vi "S4GUI_002.vi"(7 "Tab ObsEng":enum32{"Obs", "CCD modes", "Eng"}(tab)) -> ()   [LabVIEW 2018] (continued)
                    n834 = Not(x=w1534) -> (.not. x?=w1554:bool)
                    n835 = Not(x=w1533) -> (.not. x?=w1553:bool)
                    n836 = Not(x=w1532) -> (.not. x?=w1555:bool)
                    n837 = property on="Image FInal Column 2" class="DigNum (strict)"("Blinking"=w1552) -> ()  [unwired: 2 in, 2 out]
                    n838 = property on="Frame Transfer 2" class="Bool (strict)"("Blinking"=w1550) -> ()  [unwired: 2 in, 2 out]
                    n839 = property on="Vertical Clock Voltage 2" class="Ring (strict)"("Blinking"=w1551) -> ()  [unwired: 2 in, 2 out]
                    n840 = property on="A/D Channel 2" class="DigNum (strict)"("Blinking"=w1549) -> ()  [unwired: 2 in, 2 out]
                    n841 = property on="Image Initial Line 2" class="DigNum (strict)"("Blinking"=w1554) -> ()  [unwired: 2 in, 2 out]
                    n842 = property on="Image Initial Column 2" class="DigNum (strict)"("Blinking"=w1553) -> ()  [unwired: 2 in, 2 out]
                    n843 = property on="Image Final Line 2" class="DigNum (strict)"("Blinking"=w1555) -> ()  [unwired: 2 in, 2 out]
                    n844 = Not(x=w1524) -> (.not. x?=w1545:bool)
                    n845 = Not(x=w1523) -> (.not. x?=w1547:bool)
                    n846 = Not(x=w1522) -> (.not. x?=w1546:bool)
                    n847 = Not(x=w1521) -> (.not. x?=w1548:bool)
                    n848 = Not(x=w1527) -> (.not. x?=w1543:bool)
                    n849 = Not(x=w1526) -> (.not. x?=w1544:bool)
                    n850 = Not(x=w1525) -> (.not. x?=w1542:bool)
                    n851 = property on="Shutter Openning Time 2" class="DigNum (strict)"("Blinking"=w1545) -> ()  [unwired: 2 in, 2 out]
                    n852 = property on="Shutter Closing Time 2" class="DigNum (strict)"("Blinking"=w1547) -> ()  [unwired: 2 in, 2 out]
                    n853 = property on="Vertical Binning 2" class="DigNum (strict)"("Blinking"=w1546) -> ()  [unwired: 2 in, 2 out]
                    n854 = property on="Horizontal Binning 2" class="DigNum (strict)"("Blinking"=w1548) -> ()  [unwired: 2 in, 2 out]
                    n855 = property on="CCD EM Gain 2" class="DigNum (strict)"("Blinking"=w1543) -> ()  [unwired: 2 in, 2 out]
                    n856 = property on="Shutter Mode 2" class="Ring (strict)"("Blinking"=w1544) -> ()  [unwired: 2 in, 2 out]
                    n857 = property on="Shutter TTL 2" class="Ring (strict)"("Blinking"=w1542) -> ()  [unwired: 2 in, 2 out]
                    n858 = Not(x=w1520) -> (.not. x?=w1535:bool)
                    n859 = Not(x=w1516) -> (.not. x?=w1538:bool)
                    n860 = Not(x=w1515) -> (.not. x?=w1536:bool)
                    n861 = Not(x=w1514) -> (.not. x?=w1537:bool)
                    n862 = Not(x=w1519) -> (.not. x?=w1540:bool)
                    n863 = Not(x=w1518) -> (.not. x?=w1539:bool)
                    n864 = Not(x=w1517) -> (.not. x?=w1541:bool)
                    n865 = property on="Acquisition Mode 2" class="Ring (strict)"("Blinking"=w1535) -> ()  [unwired: 2 in, 2 out]
                    n866 = property on="Readout Rate 2" class="Ring (strict)"("Blinking"=w1538) -> ()  [unwired: 2 in, 2 out]
                    n867 = property on="Vertical Shift Speed 2" class="Ring (strict)"("Blinking"=w1536) -> ()  [unwired: 2 in, 2 out]
                    n868 = property on="CCD EM Mode 2" class="Ring (strict)"("Blinking"=w1537) -> ()  [unwired: 2 in, 2 out]
                    n869 = property on="Trigger Mode 2" class="Ring (strict)"("Blinking"=w1540) -> ()  [unwired: 2 in, 2 out]
                    n870 = property on="Read Mode 2" class="Ring (strict)"("Blinking"=w1539) -> ()  [unwired: 2 in, 2 out]
                    n871 = property on="Pre-amplification Gain 2" class="Ring (strict)"("Blinking"=w1541) -> ()  [unwired: 2 in, 2 out]
                  }
                }
                n872 = local read "Cameras Cluster"() -> (w1505:T7)
                n873 = Bundle By Name(cluster=w1505, "Current Configuration.Image Initial Line 2"=w1468, "Current Configuration.Image Initial Column 2"=w1466, "Current Configuration.Image Final Line 2"=w1469, "Current Configuration.Image FInal Column 2"=w1467, "Current Configuration.Vertical Binning 2"=w1472, "Current Configuration.Horizontal Binning 2"=w1503, "Current Configuration.Pre-amplification Gain 2"=w1471, "Current Configuration.CCD EM Gain 2"=w1470, "Current Configuration.Readout Rate 2"=w1465, "Current Configuration.Shutter Openning Time 2"=w1502, "Current Configuration.Shutter Closing Time 2"=w1501, "Current Configuration.Vertical Shift Speed 2"=w1500, "Current Configuration.Read Mode 2"=w1499, "Current Configuration.Vertical Clock Voltage 2"=w1498, "Current Configuration.A/D Channel 2"=w1497, "Current Configuration.Shutter Mode 2"=w1494, "Current Configuration.Shutter TTL 2"=w1495, "Current Configuration.Trigger Mode 2"=w1473, "Current Configuration.Frame Transfer 2"=w1474, "Current Configuration.Acquisition Mode 2"=w1496, "Current Configuration.CCD EM Mode 2"=w1464) -> (w1504:T7)
                n874 = local write "PA2"(w1459) -> ()
                n875 = local write "B2"(w1458) -> ()
                n876 = local write "EA2"(w1460) -> ()
                n877 = local write "SI2"(w1455) -> ()
                n878 = local write "RO2"(w1456) -> ()
                n879 = local write "G2"(w1457) -> ()
                n880 = local write "Cameras Cluster"(w1504) -> ()
                n881 = Compound Arithmetic op=AND(w1479, w1478, w1477, w1476, w1452, w1451, w1475, w1486, w1485, w1484, w1483, w1482, w1481, w1480, w1493, w1492, w1491, w1490, w1489, w1488, w1487) -> (w1450:bool)
                "CCD checked 2" <- w1450
                n882 = disable-structure shown="Disabled" {
                  disable-tunnel: w1450 -> [w1507 _]
                  frame Disabled {
                    n883 = Select(t=u32 1244955, s=w1507, f=u32 16718848) -> (s? t:f=w1510:u32)
                    n884 = property on="CCD checked 2" class="Bool (strict)"("Caption.BG Color"=w1510) -> ()  [unwired: 2 in, 2 out]
                  }
                  frame Enabled {
                  }
                }
                n885 = property on="Acquisition Mode 2" class="Ring (strict)"("DisabledEnum"=w1453) -> ()  [unwired: 2 in, 2 out]
                n886 = property on="Readout Rate 2" class="Ring (strict)"("DisabledEnum"=w1453) -> ()  [unwired: 2 in, 2 out]
                n887 = property on="Vertical Shift Speed 2" class="Ring (strict)"("DisabledEnum"=w1453) -> ()  [unwired: 2 in, 2 out]
                n888 = property on="CCD EM Mode 2" class="Ring (strict)"("DisabledEnum"=w1453) -> ()  [unwired: 2 in, 2 out]
                n889 = property on="Shutter Openning Time 2" class="DigNum (strict)"("DisabledEnum"=w1453) -> ()  [unwired: 2 in, 2 out]
                n890 = property on="Shutter Closing Time 2" class="DigNum (strict)"("DisabledEnum"=w1453) -> ()  [unwired: 2 in, 2 out]
                n891 = property on="Vertical Binning 2" class="DigNum (strict)"("DisabledEnum"=w1453) -> ()  [unwired: 2 in, 2 out]
                n892 = property on="Horizontal Binning 2" class="DigNum (strict)"("DisabledEnum"=w1453) -> ()  [unwired: 2 in, 2 out]
                n893 = property on="Trigger Mode 2" class="Ring (strict)"("DisabledEnum"=w1453) -> ()  [unwired: 2 in, 2 out]
                n894 = property on="Read Mode 2" class="Ring (strict)"("DisabledEnum"=w1453) -> ()  [unwired: 2 in, 2 out]
                n895 = property on="Pre-amplification Gain 2" class="Ring (strict)"("DisabledEnum"=w1453) -> ()  [unwired: 2 in, 2 out]
                n896 = property on="CCD EM Gain 2" class="DigNum (strict)"("DisabledEnum"=w1453) -> ()  [unwired: 2 in, 2 out]
                n897 = property on="Shutter Mode 2" class="Ring (strict)"("DisabledEnum"=w1453) -> ()  [unwired: 2 in, 2 out]
                n898 = property on="Shutter TTL 2" class="Ring (strict)"("DisabledEnum"=w1453) -> ()  [unwired: 2 in, 2 out]
                n899 = property on="Image FInal Column 2" class="DigNum (strict)"("DisabledEnum"=w1453) -> ()  [unwired: 2 in, 2 out]
                n900 = property on="Frame Transfer 2" class="Bool (strict)"("DisabledEnum"=w1453) -> ()  [unwired: 2 in, 2 out]
                n901 = property on="Vertical Clock Voltage 2" class="Ring (strict)"("DisabledEnum"=w1453) -> ()  [unwired: 2 in, 2 out]
                n902 = property on="A/D Channel 2" class="DigNum (strict)"("DisabledEnum"=w1453) -> ()  [unwired: 2 in, 2 out]
                n903 = property on="Image Initial Line 2" class="DigNum (strict)"("DisabledEnum"=w1453) -> ()  [unwired: 2 in, 2 out]
                n904 = property on="Image Initial Column 2" class="DigNum (strict)"("DisabledEnum"=w1453) -> ()  [unwired: 2 in, 2 out]
                n905 = property on="Image Final Line 2" class="DigNum (strict)"("DisabledEnum"=w1453) -> ()  [unwired: 2 in, 2 out]
              }
              frame #17 {
                # "Carrega coluna do Channel 3"
                # "Aba:  Eng->Camera"
                n906 = Unbundle By Name(w1669) -> ("ChannelC_CCD"=w1639:T29, "CHC_Checked Params"=w1654:T14, "ChannelC_Status.connection"=w1632:bool)
                n907 = Unbundle By Name(w1654) -> ("ACQUISITION_MODE"=w1621:bool, "TRIGGER_MODE"=w1620:bool, "READ_MODE"=w1619:bool, "PREAMP"=w1618:bool, "READOUT_RATE"=w1617:bool, "VERTICAL_SHIFT_SPEED"=w1616:bool, "EM_MODE"=w1615:bool, "EM_GAIN"=w1652:bool, "SHUTTER_MODE"=w1651:bool, "SHUTTER_TTL"=w1650:bool, "SHUTTER_OPENING_TIME"=w1649:bool, "SHUTTER_CLOSING_TIME"=w1631:bool, "VBIN"=w1623:bool, "HBIN"=w1622:bool, "INITIAL_LINE"=w1630:bool, "INITIAL_COLUMN"=w1629:bool, "FINAL_LINE"=w1628:bool, "FINAL_COLUMN"=w1627:bool, "FRAME_TRANSFER"=w1626:bool, "VERTICAL_CLOCK_VOLTAGE"=w1625:bool, "AD_CHANNEL"=w1624:bool)
                n908 = case shown="True" w1632 {
                  tunnel: w1639 -> [_ w1722]
                  tunnel: [w1715 w1721] -> w1638
                  tunnel: [w1715 w1720] -> w1637
                  tunnel: [w1715 w1719] -> w1636
                  tunnel: [w1715 w1718] -> w1635
                  tunnel: [w1715 w1717] -> w1634
                  tunnel: [w1715 w1716] -> w1633
                  frame False {
                    w1715 = ""
                  }
                  frame True {
                    n909 = stacked-sequence "Atualizacao dos indicadores inferiores do CANAL C da tela principal" {
                      tunnel: w1722 -> [w1737 w1740 w1745 w1754 w1757 w1761]
                      tunnel: [w1723 _ _ _ _ _] -> w1721
                      tunnel: [_ w1738 _ _ _ _] -> w1720
                      tunnel: [_ _ w1743 _ _ _] -> w1719
                      tunnel: [_ _ _ w1748 _ _] -> w1718
                      tunnel: [_ _ _ _ w1755 _] -> w1717
                      tunnel: [_ _ _ _ _ w1758] -> w1716
                      frame #0 {
                        # "SubImage"
                        n910 = Unbundle By Name(w1737) -> ("INITIAL_LINE"=w1735:u16, "FINAL_LINE"=w1734:u16, "INITIAL_COLUMN"=w1733:u16, "FINAL_COLUMN"=w1732:u16)
                        n911 = Number To Decimal String(number=w1735) -> (decimal integer string=w1731:string)  [unwired: 1 in]
                        n912 = Number To Decimal String(number=w1734) -> (decimal integer string=w1729:string)  [unwired: 1 in]
                        n913 = Number To Decimal String(number=w1733) -> (decimal integer string=w1727:string)  [unwired: 1 in]
                        n914 = Number To Decimal String(number=w1732) -> (decimal integer string=w1725:string)  [unwired: 1 in]
                        n915 = Concatenate Strings("[", w1731, ":", w1729, ",", w1727, ":", w1725, "]") -> (w1723:string)
                      }
                      frame #1 {
                        # "Em Active"
                        n916 = Unbundle By Name(w1740) -> ("EM_MODE"=w1739:u8)
                        n917 = case shown="0, Default" w1739 {
                          tunnel: ["Electron M." ("EmActive1") "Convent." ("EmActive1")] -> w1738
                          frame 0, Default {
                          }
                          frame 1 {
                          }
                        }
                      }
                      frame #2 {
                        # "Pre Amp"
                        n918 = Unbundle By Name(w1745) -> ("PREAMP"=w1744:u8)
                        n919 = case shown="1" w1744 {
                          tunnel: ["Gain 1" ("EmActive1") "Gain 2" ("EmActive1")] -> w1743
                          frame 0, Default {
                          }
                          frame 1 {
                          }
                        }
                      }
                      frame #3 {
                        # "Binning"
                        n920 = Unbundle By Name(w1754) -> ("VBIN"=w1753:u16, "HBIN"=w1752:u16)
                        n921 = Number To Decimal String(number=w1752) -> (decimal integer string=w1749:string)  [unwired: 1 in]
                        n922 = Number To Decimal String(number=w1753) -> (decimal integer string=w1751:string)  [unwired: 1 in]
                        n923 = Concatenate Strings(w1751, "x", w1749) -> (w1748:string)
                      }
                      frame #4 {
                        # "Gain"
                        n924 = Unbundle By Name(w1757) -> ("EM_GAIN"=w1756:u16)
                        n925 = Number To Decimal String(number=w1756) -> (decimal integer string=w1755:string)  [unwired: 1 in]
                      }
                      frame #5 {
                        # "Readout"
                        n926 = Unbundle By Name(w1761) -> ("EM_MODE"=w1760:u8, "READOUT_RATE"=w1759:u8)
                        n927 = case shown="0, Default" w1760 {
                          tunnel: w1759 -> [w1763 w1769]
                          tunnel: [w1762 w1768] -> w1758
                          frame 0, Default {
                            n928 = case shown="3" w1763 {
                              tunnel: ["30 MHz" ("EmActive1") "20 MHz" ("EmActive1") "10 MHz" ("EmActive1") "1 MHz" ("EmActive1")] -> w1762
                              frame 0, Default {
                              }
                              frame 1 {
                              }
                              frame 2 {
                              }
                              frame 3 {
                              }
                            }
                          }
                          frame 1 {
                            n929 = case shown="1" w1769 {
                              tunnel: ["1 MHz" ("EmActive1") "0.1 MHz" ("EmActive1")] -> w1768
                              frame 0, Default {
                              }
                              frame 1 {
                              }
                            }
                          }
                        }
                      }
                    }
                  }
                }
                n930 = Unbundle By Name(w1639) -> ("INITIAL_LINE"=w1644:u16, "INITIAL_COLUMN"=w1642:u16, "FINAL_LINE"=w1645:u16, "FINAL_COLUMN"=w1643:u16, "VBIN"=w1648:u16, "HBIN"=w1666:u16, "PREAMP"=w1647:u8, "EM_GAIN"=w1646:u16, "READOUT_RATE"=w1641:u8, "SHUTTER_OPENNING_TIME"=w1665:u16, "SHUTTER_CLOSING_TIME"=w1664:u16, "VERTICAL_SHIFT_SPEED"=w1663:u8, "READ_MODE"=w1662:u8, "VERTICAL_CLOCK_VOLTAGE"=w1661:u8, "AD_CHANNEL"=w1660:u32, "SHUTTER_MODE"=w1655:u8, "SHUTTER_TTL"=w1656:u8, "TRIGGER_MODE"=w1657:u8, "FRAME_TRANSFER"=w1658:bool, "ACQUISITION_MODE"=w1659:u8, "EM_MODE"=w1640:u8)
                n931 = local read "CH3 on"() -> (w1614:bool)
                n932 = case shown="True" w1614 {
                  tunnel: w1652 -> [_ w1695]
                  tunnel: w1651 -> [_ w1694]
                  tunnel: w1650 -> [_ w1692]
                  tunnel: w1649 -> [_ w1691]
                  tunnel: w1631 -> [_ w1690]
                  tunnel: w1630 -> [_ w1689]
                  tunnel: w1629 -> [_ w1688]
                  tunnel: w1628 -> [_ w1687]
                  tunnel: w1627 -> [_ w1686]
                  tunnel: w1626 -> [_ w1685]
                  tunnel: w1625 -> [_ w1684]
                  tunnel: w1624 -> [_ w1683]
                  tunnel: w1623 -> [_ w1682]
                  tunnel: w1622 -> [_ w1681]
                  tunnel: w1621 -> [_ w1680]
                  tunnel: w1620 -> [_ w1679]
                  tunnel: w1619 -> [_ w1678]
                  tunnel: w1618 -> [_ w1677]
                  tunnel: w1617 -> [_ w1676]
                  tunnel: w1616 -> [_ w1675]
                  tunnel: w1615 -> [_ w1674]
                  tunnel: [T12."Disabled and Grayed Out" ("Disabled") T12."Enabled" ("Disabled")] -> w1613
                  frame False {
                    w1670 = FALSE
                    n933 = property on="Image Initial Line 3" class="DigNum (strict)"("Blinking"=w1670) -> ()  [unwired: 2 in, 2 out]
                    n934 = property on="Image Initial Column 3" class="DigNum (strict)"("Blinking"=w1670) -> ()  [unwired: 2 in, 2 out]
                    n935 = property on="Image Final Line 3" class="DigNum (strict)"("Blinking"=w1670) -> ()  [unwired: 2 in, 2 out]
                    n936 = property on="Image FInal Column 3" class="DigNum (strict)"("Blinking"=w1670) -> ()  [unwired: 2 in, 2 out]
                    n937 = property on="Frame Transfer 3" class="Bool (strict)"("Blinking"=w1670) -> ()  [unwired: 2 in, 2 out]
                    n938 = property on="Vertical Clock Voltage 3" class="Ring (strict)"("Blinking"=w1670) -> ()  [unwired: 2 in, 2 out]
                    n939 = property on="A/D Channel 3" class="DigNum (strict)"("Blinking"=w1670) -> ()  [unwired: 2 in, 2 out]
                    n940 = property on="CCD EM Gain 3" class="DigNum (strict)"("Blinking"=w1670) -> ()  [unwired: 2 in, 2 out]
                    n941 = property on="Shutter Mode 3" class="Ring (strict)"("Blinking"=w1670) -> ()  [unwired: 2 in, 2 out]
                    n942 = property on="Shutter TTL 3" class="Ring (strict)"("Blinking"=w1670) -> ()  [unwired: 2 in, 2 out]
                    n943 = property on="Shutter Openning Time 3" class="DigNum (strict)"("Blinking"=w1670) -> ()  [unwired: 2 in, 2 out]
                    n944 = property on="Shutter Closing Time 3" class="DigNum (strict)"("Blinking"=w1670) -> ()  [unwired: 2 in, 2 out]
                    n945 = property on="Vertical Binning 3" class="DigNum (strict)"("Blinking"=w1670) -> ()  [unwired: 2 in, 2 out]
                    n946 = property on="Horizontal Binning 3" class="DigNum (strict)"("Blinking"=w1670) -> ()  [unwired: 2 in, 2 out]
                    n947 = property on="Acquisition Mode 3" class="Ring (strict)"("Blinking"=w1670) -> ()  [unwired: 2 in, 2 out]
                    n948 = property on="Vertical Shift Speed 3" class="Ring (strict)"("Blinking"=w1670) -> ()  [unwired: 2 in, 2 out]
                    n949 = property on="Trigger Mode 3" class="Ring (strict)"("Blinking"=w1670) -> ()  [unwired: 2 in, 2 out]
                    n950 = property on="Read Mode 3" class="Ring (strict)"("Blinking"=w1670) -> ()  [unwired: 2 in, 2 out]
                    n951 = property on="Readout Rate 3" class="Ring (strict)"("Blinking"=w1670) -> ()  [unwired: 2 in, 2 out]
                    n952 = property on="CCD EM Mode 3" class="Ring (strict)"("Blinking"=w1670) -> ()  [unwired: 2 in, 2 out]
                    n953 = property on="Pre-amplification Gain 3" class="Ring (strict)"("Blinking"=w1670) -> ()  [unwired: 2 in, 2 out]
                  }
                  frame True {
                    n954 = Not(x=w1689) -> (.not. x?=w1672:bool)
                    n955 = Not(x=w1688) -> (.not. x?=w1713:bool)
                    n956 = Not(x=w1687) -> (.not. x?=w1714:bool)
                    n957 = Not(x=w1686) -> (.not. x?=w1712:bool)
                    n958 = Not(x=w1685) -> (.not. x?=w1710:bool)
                    n959 = Not(x=w1684) -> (.not. x?=w1711:bool)
                    n960 = Not(x=w1683) -> (.not. x?=w1709:bool)
                    n961 = property on="Image FInal Column 3" class="DigNum (strict)"("Blinking"=w1712) -> ()  [unwired: 2 in, 2 out]
                    n962 = property on="Frame Transfer 3" class="Bool (strict)"("Blinking"=w1710) -> ()  [unwired: 2 in, 2 out]
                    n963 = property on="Vertical Clock Voltage 3" class="Ring (strict)"("Blinking"=w1711) -> ()  [unwired: 2 in, 2 out]
                    n964 = property on="Image Initial Line 3" class="DigNum (strict)"("Blinking"=w1672) -> ()  [unwired: 2 in, 2 out]
                    n965 = property on="Image Initial Column 3" class="DigNum (strict)"("Blinking"=w1713) -> ()  [unwired: 2 in, 2 out]
                    n966 = property on="Image Final Line 3" class="DigNum (strict)"("Blinking"=w1714) -> ()  [unwired: 2 in, 2 out]
                    n967 = property on="A/D Channel 3" class="DigNum (strict)"("Blinking"=w1709) -> ()  [unwired: 2 in, 2 out]
                    n968 = Not(x=w1691) -> (.not. x?=w1705:bool)
                    n969 = Not(x=w1690) -> (.not. x?=w1707:bool)
                    n970 = Not(x=w1682) -> (.not. x?=w1706:bool)
                    n971 = Not(x=w1681) -> (.not. x?=w1708:bool)
                    n972 = Not(x=w1695) -> (.not. x?=w1704:bool)
                    n973 = Not(x=w1694) -> (.not. x?=w1693:bool)
                    n974 = Not(x=w1692) -> (.not. x?=w1703:bool)
                    n975 = property on="Shutter Openning Time 3" class="DigNum (strict)"("Blinking"=w1705) -> ()  [unwired: 2 in, 2 out]
                    n976 = property on="Shutter Closing Time 3" class="DigNum (strict)"("Blinking"=w1707) -> ()  [unwired: 2 in, 2 out]
                    n977 = property on="Vertical Binning 3" class="DigNum (strict)"("Blinking"=w1706) -> ()  [unwired: 2 in, 2 out]
                    n978 = property on="Horizontal Binning 3" class="DigNum (strict)"("Blinking"=w1708) -> ()  [unwired: 2 in, 2 out]
                    n979 = property on="CCD EM Gain 3" class="DigNum (strict)"("Blinking"=w1704) -> ()  [unwired: 2 in, 2 out]
                    n980 = property on="Shutter Mode 3" class="Ring (strict)"("Blinking"=w1693) -> ()  [unwired: 2 in, 2 out]
                    n981 = property on="Shutter TTL 3" class="Ring (strict)"("Blinking"=w1703) -> ()  [unwired: 2 in, 2 out]
                    n982 = Not(x=w1680) -> (.not. x?=w1696:bool)
                    n983 = Not(x=w1676) -> (.not. x?=w1699:bool)
                    n984 = Not(x=w1675) -> (.not. x?=w1697:bool)
                    n985 = Not(x=w1674) -> (.not. x?=w1698:bool)
                    n986 = Not(x=w1679) -> (.not. x?=w1701:bool)
                    n987 = Not(x=w1678) -> (.not. x?=w1700:bool)
                    n988 = Not(x=w1677) -> (.not. x?=w1702:bool)
                    n989 = property on="Acquisition Mode 3" class="Ring (strict)"("Blinking"=w1696) -> ()  [unwired: 2 in, 2 out]
                    n990 = property on="Readout Rate 3" class="Ring (strict)"("Blinking"=w1699) -> ()  [unwired: 2 in, 2 out]
                    n991 = property on="Vertical Shift Speed 3" class="Ring (strict)"("Blinking"=w1697) -> ()  [unwired: 2 in, 2 out]
                    n992 = property on="CCD EM Mode 3" class="Ring (strict)"("Blinking"=w1698) -> ()  [unwired: 2 in, 2 out]
                    n993 = property on="Trigger Mode 3" class="Ring (strict)"("Blinking"=w1701) -> ()  [unwired: 2 in, 2 out]
                    n994 = property on="Read Mode 3" class="Ring (strict)"("Blinking"=w1700) -> ()  [unwired: 2 in, 2 out]
                    n995 = property on="Pre-amplification Gain 3" class="Ring (strict)"("Blinking"=w1702) -> ()  [unwired: 2 in, 2 out]
                  }
                }
                n996 = local write "RO3"(w1633) -> ()
                n997 = local write "B3"(w1635) -> ()
                n998 = local write "PA3"(w1636) -> ()
                n999 = local write "EA3"(w1637) -> ()
                n1000 = local write "G3"(w1634) -> ()
                n1001 = local write "SI3"(w1638) -> ()
                n1002 = local read "Cameras Cluster"() -> (w1668:T7)
                n1003 = Bundle By Name(cluster=w1668, "Current Configuration.Image Initial Line 3"=w1644, "Current Configuration.Image Initial Column 3"=w1642, "Current Configuration.Image Final Line 3"=w1645, "Current Configuration.Image FInal Column 3"=w1643, "Current Configuration.Vertical Binning 3"=w1648, "Current Configuration.Horizontal Binning 3"=w1666, "Current Configuration.Pre-amplification Gain 3"=w1647, "Current Configuration.CCD EM Gain 3"=w1646, "Current Configuration.Readout Rate 3"=w1641, "Current Configuration.Shutter Openning Time 3"=w1665, "Current Configuration.Shutter Closing Time 3"=w1664, "Current Configuration.Vertical Shift Speed 3"=w1663, "Current Configuration.Read Mode 3"=w1662, "Current Configuration.Vertical Clock Voltage 3"=w1661, "Current Configuration.A/D Channel 3"=w1660, "Current Configuration.Shutter Mode 3"=w1655, "Current Configuration.Shutter TTL 3"=w1656, "Current Configuration.Trigger Mode 3"=w1657, "Current Configuration.Frame Transfer 3"=w1658, "Current Configuration.Acquisition Mode 3"=w1659, "Current Configuration.CCD EM Mode 3"=w1640) -> (w1667:T7)
                n1004 = local write "Cameras Cluster"(w1667) -> ()
                n1005 = Compound Arithmetic op=AND(w1621, w1620, w1619, w1618, w1617, w1616, w1615, w1652, w1651, w1650, w1649, w1631, w1623, w1622, w1630, w1629, w1628, w1627, w1626, w1625, w1624) -> (→"CCD checked 3":bool)
                n1006 = property on="Image Initial Line 3" class="DigNum (strict)"("DisabledEnum"=w1613) -> ()  [unwired: 2 in, 2 out]
                n1007 = property on="Image Initial Column 3" class="DigNum (strict)"("DisabledEnum"=w1613) -> ()  [unwired: 2 in, 2 out]
                n1008 = property on="Image Final Line 3" class="DigNum (strict)"("DisabledEnum"=w1613) -> ()  [unwired: 2 in, 2 out]
                n1009 = property on="Image FInal Column 3" class="DigNum (strict)"("DisabledEnum"=w1613) -> ()  [unwired: 2 in, 2 out]
                n1010 = property on="Frame Transfer 3" class="Bool (strict)"("DisabledEnum"=w1613) -> ()  [unwired: 2 in, 2 out]
                n1011 = property on="Horizontal Binning 3" class="DigNum (strict)"("DisabledEnum"=w1613) -> ()  [unwired: 2 in, 2 out]
                n1012 = property on="Vertical Clock Voltage 3" class="Ring (strict)"("DisabledEnum"=w1613) -> ()  [unwired: 2 in, 2 out]
                n1013 = property on="CCD EM Gain 3" class="DigNum (strict)"("DisabledEnum"=w1613) -> ()  [unwired: 2 in, 2 out]
                n1014 = property on="Shutter Mode 3" class="Ring (strict)"("DisabledEnum"=w1613) -> ()  [unwired: 2 in, 2 out]
                n1015 = property on="Shutter Openning Time 3" class="DigNum (strict)"("DisabledEnum"=w1613) -> ()  [unwired: 2 in, 2 out]
                n1016 = property on="Shutter Closing Time 3" class="DigNum (strict)"("DisabledEnum"=w1613) -> ()  [unwired: 2 in, 2 out]
                n1017 = property on="Vertical Binning 3" class="DigNum (strict)"("DisabledEnum"=w1613) -> ()  [unwired: 2 in, 2 out]
                n1018 = property on="Shutter TTL 3" class="Ring (strict)"("DisabledEnum"=w1613) -> ()  [unwired: 2 in, 2 out]
                n1019 = property on="Pre-amplification Gain 3" class="Ring (strict)"("DisabledEnum"=w1613) -> ()  [unwired: 2 in, 2 out]
                n1020 = property on="Acquisition Mode 3" class="Ring (strict)"("DisabledEnum"=w1613) -> ()  [unwired: 2 in, 2 out]
                n1021 = property on="Trigger Mode 3" class="Ring (strict)"("DisabledEnum"=w1613) -> ()  [unwired: 2 in, 2 out]
                n1022 = property on="Read Mode 3" class="Ring (strict)"("DisabledEnum"=w1613) -> ()  [unwired: 2 in, 2 out]
                n1023 = property on="Readout Rate 3" class="Ring (strict)"("DisabledEnum"=w1613) -> ()  [unwired: 2 in, 2 out]
                n1024 = property on="A/D Channel 3" class="DigNum (strict)"("DisabledEnum"=w1613) -> ()  [unwired: 2 in, 2 out]
                n1025 = property on="Vertical Shift Speed 3" class="Ring (strict)"("DisabledEnum"=w1613) -> ()  [unwired: 2 in, 2 out]
                n1026 = property on="CCD EM Mode 3" class="Ring (strict)"("DisabledEnum"=w1613) -> ()  [unwired: 2 in, 2 out]
              }
              frame #18 {
                # "Carrega coluna do Channel 4"
                # "Aba:  Eng->Camera"
                n1027 = Unbundle By Name(w1828) -> ("ChannelD_CCD"=w1781:T29, "CHD_Checked Params"=w1813:T14, "ChannelD_Status.connection"=w1780:bool)
                n1028 = Unbundle By Name(w1813) -> ("ACQUISITION_MODE"=w1797:bool, "TRIGGER_MODE"=w1796:bool, "READ_MODE"=w1795:bool, "PREAMP"=w1794:bool, "READOUT_RATE"=w1793:bool, "VERTICAL_SHIFT_SPEED"=w1792:bool, "EM_MODE"=w1791:bool, "EM_GAIN"=w1804:bool, "SHUTTER_MODE"=w1803:bool, "SHUTTER_TTL"=w1802:bool, "SHUTTER_OPENING_TIME"=w1801:bool, "SHUTTER_CLOSING_TIME"=w1800:bool, "VBIN"=w1799:bool, "HBIN"=w1798:bool, "INITIAL_LINE"=w1811:bool, "INITIAL_COLUMN"=w1810:bool, "FINAL_LINE"=w1809:bool, "FINAL_COLUMN"=w1808:bool, "FRAME_TRANSFER"=w1807:bool, "VERTICAL_CLOCK_VOLTAGE"=w1806:bool, "AD_CHANNEL"=w1805:bool)
                n1029 = case shown="True" w1780 {
                  tunnel: w1781 -> [_ w1881]
                  tunnel: [w1874 w1880] -> w1779
                  tunnel: [w1874 w1879] -> w1778
                  tunnel: [w1874 w1878] -> w1777
                  tunnel: [w1874 w1877] -> w1776
                  tunnel: [w1874 w1876] -> w1775
                  tunnel: [w1874 w1875] -> w1774
                  frame False {
                    w1874 = ""
                  }
                  frame True {
                    n1030 = stacked-sequence "Atualizacao dos indicadores inferiores do CANAL D da tela principal" {
                      tunnel: w1881 -> [w1896 w1899 w1904 w1913 w1916 w1920]
                      tunnel: [w1882 _ _ _ _ _] -> w1880
                      tunnel: [_ w1897 _ _ _ _] -> w1879
                      tunnel: [_ _ w1902 _ _ _] -> w1878
                      tunnel: [_ _ _ w1907 _ _] -> w1877
                      tunnel: [_ _ _ _ w1914 _] -> w1876
                      tunnel: [_ _ _ _ _ w1917] -> w1875
                      frame #0 {
                        # "SubImage"
                        n1031 = Unbundle By Name(w1896) -> ("INITIAL_LINE"=w1894:u16, "FINAL_LINE"=w1893:u16, "INITIAL_COLUMN"=w1892:u16, "FINAL_COLUMN"=w1891:u16)
                        n1032 = Number To Decimal String(number=w1894) -> (decimal integer string=w1890:string)  [unwired: 1 in]
                        n1033 = Number To Decimal String(number=w1893) -> (decimal integer string=w1888:string)  [unwired: 1 in]
                        n1034 = Number To Decimal String(number=w1892) -> (decimal integer string=w1886:string)  [unwired: 1 in]
                        n1035 = Number To Decimal String(number=w1891) -> (decimal integer string=w1884:string)  [unwired: 1 in]
                        n1036 = Concatenate Strings("[", w1890, ":", w1888, ",", w1886, ":", w1884, "]") -> (w1882:string)
                      }
                      frame #1 {
                        # "Em Active"
                        n1037 = Unbundle By Name(w1899) -> ("EM_MODE"=w1898:u8)
                        n1038 = case shown="0, Default" w1898 {
                          tunnel: ["Electron M." ("EmActive1") "Convent." ("EmActive1")] -> w1897
                          frame 0, Default {
                          }
                          frame 1 {
                          }
                        }
                      }
                      frame #2 {
                        # "Pre Amp"
                        n1039 = Unbundle By Name(w1904) -> ("PREAMP"=w1903:u8)
                        n1040 = case shown="1" w1903 {
                          tunnel: ["Gain 1" ("EmActive1") "Gain 2" ("EmActive1")] -> w1902
                          frame 0, Default {
                          }
                          frame 1 {
                          }
                        }
                      }
                      frame #3 {
                        # "Binning"
                        n1041 = Unbundle By Name(w1913) -> ("VBIN"=w1912:u16, "HBIN"=w1911:u16)
                        n1042 = Number To Decimal String(number=w1911) -> (decimal integer string=w1908:string)  [unwired: 1 in]
                        n1043 = Number To Decimal String(number=w1912) -> (decimal integer string=w1910:string)  [unwired: 1 in]
                        n1044 = Concatenate Strings(w1910, "x", w1908) -> (w1907:string)
                      }
                      frame #4 {
                        # "Gain"
                        n1045 = Unbundle By Name(w1916) -> ("EM_GAIN"=w1915:u16)
                        n1046 = Number To Decimal String(number=w1915) -> (decimal integer string=w1914:string)  [unwired: 1 in]
                      }
                      frame #5 {
                        # "Readout"
                        n1047 = Unbundle By Name(w1920) -> ("EM_MODE"=w1919:u8, "READOUT_RATE"=w1918:u8)
                        n1048 = case shown="0, Default" w1919 {
                          tunnel: w1918 -> [w1922 w1928]
                          tunnel: [w1921 w1927] -> w1917
                          frame 0, Default {
                            n1049 = case shown="3" w1922 {
                              tunnel: ["30 MHz" ("EmActive1") "20 MHz" ("EmActive1") "10 MHz" ("EmActive1") "1 MHz" ("EmActive1")] -> w1921
                              frame 0, Default {
                              }
                              frame 1 {
                              }
                              frame 2 {
                              }
                              frame 3 {
                              }
                            }
                          }
                          frame 1 {
                            n1050 = case shown="0, Default" w1928 {
                              tunnel: ["1 MHz" ("EmActive1") "0.1 MHz" ("EmActive1")] -> w1927
                              frame 0, Default {
                              }
                              frame 1 {
                              }
                            }
                          }
                        }
                      }
                    }
                  }
                }
                n1051 = Unbundle By Name(w1781) -> ("INITIAL_LINE"=w1786:u16, "INITIAL_COLUMN"=w1784:u16, "FINAL_LINE"=w1787:u16, "FINAL_COLUMN"=w1785:u16, "VBIN"=w1790:u16, "HBIN"=w1825:u16, "PREAMP"=w1789:u8, "EM_GAIN"=w1788:u16, "READOUT_RATE"=w1783:u8, "SHUTTER_OPENNING_TIME"=w1824:u16, "SHUTTER_CLOSING_TIME"=w1823:u16, "VERTICAL_SHIFT_SPEED"=w1822:u8, "READ_MODE"=w1821:u8, "VERTICAL_CLOCK_VOLTAGE"=w1820:u8, "AD_CHANNEL"=w1819:u32, "SHUTTER_MODE"=w1814:u8, "SHUTTER_TTL"=w1815:u8, "TRIGGER_MODE"=w1816:u8, "FRAME_TRANSFER"=w1817:bool, "ACQUISITION_MODE"=w1818:u8, "EM_MODE"=w1782:u8)
                n1052 = local read "CH4 on"() -> (w1773:bool)
                n1053 = case shown="False" w1773 {
                  tunnel: w1811 -> [_ w1853]
                  tunnel: w1810 -> [_ w1852]
                  tunnel: w1809 -> [_ w1851]
                  tunnel: w1808 -> [_ w1850]
                  tunnel: w1807 -> [_ w1849]
                  tunnel: w1806 -> [_ w1848]
                  tunnel: w1805 -> [_ w1847]
                  tunnel: w1804 -> [_ w1846]
                  tunnel: w1803 -> [_ w1845]
                  tunnel: w1802 -> [_ w1844]
                  tunnel: w1801 -> [_ w1843]
                  tunnel: w1800 -> [_ w1842]
                  tunnel: w1799 -> [_ w1841]
                  tunnel: w1798 -> [_ w1840]
                  tunnel: w1797 -> [_ w1839]
                  tunnel: w1796 -> [_ w1838]
                  tunnel: w1795 -> [_ w1837]
                  tunnel: w1794 -> [_ w1835]
                  tunnel: w1793 -> [_ w1834]
                  tunnel: w1792 -> [_ w1833]
                  tunnel: w1791 -> [_ w1832]
                  tunnel: [T12."Disabled and Grayed Out" ("Disabled") T12."Enabled" ("Disabled")] -> w1772
                  frame False {
                    w1830 = FALSE ("Blinking")
                    n1054 = property on="Image FInal Column 4" class="DigNum (strict)"("Blinking"=w1830) -> ()  [unwired: 2 in, 2 out]
                    n1055 = property on="Frame Transfer 4" class="Bool (strict)"("Blinking"=w1830) -> ()  [unwired: 2 in, 2 out]
                    n1056 = property on="Vertical Clock Voltage 4" class="Ring (strict)"("Blinking"=w1830) -> ()  [unwired: 2 in, 2 out]
                    n1057 = property on="A/D Channel 4" class="DigNum (strict)"("Blinking"=w1830) -> ()  [unwired: 2 in, 2 out]
                    n1058 = property on="Image Initial Line 4" class="DigNum (strict)"("Blinking"=w1830) -> ()  [unwired: 2 in, 2 out]
                    n1059 = property on="Image Initial Column 4" class="DigNum (strict)"("Blinking"=w1830) -> ()  [unwired: 2 in, 2 out]
                    n1060 = property on="Image Final Line 4" class="DigNum (strict)"("Blinking"=w1830) -> ()  [unwired: 2 in, 2 out]
                    n1061 = property on="Shutter Openning Time 4" class="DigNum (strict)"("Blinking"=w1830) -> ()  [unwired: 2 in, 2 out]
                    n1062 = property on="Shutter Closing Time 4" class="DigNum (strict)"("Blinking"=w1830) -> ()  [unwired: 2 in, 2 out]
                    n1063 = property on="Vertical Binning 4" class="DigNum (strict)"("Blinking"=w1830) -> ()  [unwired: 2 in, 2 out]
                    n1064 = property on="Horizontal Binning 4" class="DigNum (strict)"("Blinking"=w1830) -> ()  [unwired: 2 in, 2 out]
                    n1065 = property on="CCD EM Gain 4" class="DigNum (strict)"("Blinking"=w1830) -> ()  [unwired: 2 in, 2 out]
                    n1066 = property on="Shutter Mode 4" class="Ring (strict)"("Blinking"=w1830) -> ()  [unwired: 2 in, 2 out]
                    n1067 = property on="Shutter TTL 4" class="Ring (strict)"("Blinking"=w1830) -> ()  [unwired: 2 in, 2 out]
                    n1068 = property on="Acquisition Mode 4" class="Ring (strict)"("Blinking"=w1830) -> ()  [unwired: 2 in, 2 out]
                    n1069 = property on="Readout Rate 4" class="Ring (strict)"("Blinking"=w1830) -> ()  [unwired: 2 in, 2 out]
                    n1070 = property on="Vertical Shift Speed 4" class="Ring (strict)"("Blinking"=w1830) -> ()  [unwired: 2 in, 2 out]
                    n1071 = property on="CCD EM Mode 4" class="Ring (strict)"("Blinking"=w1830) -> ()  [unwired: 2 in, 2 out]
                    n1072 = property on="Trigger Mode 4" class="Ring (strict)"("Blinking"=w1830) -> ()  [unwired: 2 in, 2 out]
                    n1073 = property on="Read Mode 4" class="Ring (strict)"("Blinking"=w1830) -> ()  [unwired: 2 in, 2 out]
                    n1074 = property on="Pre-amplification Gain 4" class="Ring (strict)"("Blinking"=w1830) -> ()  [unwired: 2 in, 2 out]
                  }
                  frame True {
                    n1075 = Not(x=w1850) -> (.not. x?=w1870:bool)
                    n1076 = Not(x=w1849) -> (.not. x?=w1868:bool)
                    n1077 = Not(x=w1848) -> (.not. x?=w1869:bool)
                    n1078 = Not(x=w1847) -> (.not. x?=w1867:bool)
                    n1079 = Not(x=w1853) -> (.not. x?=w1872:bool)
                    n1080 = Not(x=w1852) -> (.not. x?=w1871:bool)
                    n1081 = Not(x=w1851) -> (.not. x?=w1873:bool)
                    n1082 = property on="Image FInal Column 4" class="DigNum (strict)"("Blinking"=w1870) -> ()  [unwired: 2 in, 2 out]
                    n1083 = property on="Frame Transfer 4" class="Bool (strict)"("Blinking"=w1868) -> ()  [unwired: 2 in, 2 out]
                    n1084 = property on="Vertical Clock Voltage 4" class="Ring (strict)"("Blinking"=w1869) -> ()  [unwired: 2 in, 2 out]
                    n1085 = property on="A/D Channel 4" class="DigNum (strict)"("Blinking"=w1867) -> ()  [unwired: 2 in, 2 out]
                    n1086 = property on="Image Initial Line 4" class="DigNum (strict)"("Blinking"=w1872) -> ()  [unwired: 2 in, 2 out]
                    n1087 = property on="Image Initial Column 4" class="DigNum (strict)"("Blinking"=w1871) -> ()  [unwired: 2 in, 2 out]
                    n1088 = property on="Image Final Line 4" class="DigNum (strict)"("Blinking"=w1873) -> ()  [unwired: 2 in, 2 out]
                    n1089 = Not(x=w1843) -> (.not. x?=w1863:bool)
                    n1090 = Not(x=w1842) -> (.not. x?=w1865:bool)
                    n1091 = Not(x=w1841) -> (.not. x?=w1864:bool)
                    n1092 = Not(x=w1840) -> (.not. x?=w1866:bool)
                    n1093 = Not(x=w1846) -> (.not. x?=w1861:bool)
                    n1094 = Not(x=w1845) -> (.not. x?=w1862:bool)
                    n1095 = Not(x=w1844) -> (.not. x?=w1860:bool)
                    n1096 = property on="Shutter Openning Time 4" class="DigNum (strict)"("Blinking"=w1863) -> ()  [unwired: 2 in, 2 out]
                    n1097 = property on="Shutter Closing Time 4" class="DigNum (strict)"("Blinking"=w1865) -> ()  [unwired: 2 in, 2 out]
                    n1098 = property on="Vertical Binning 4" class="DigNum (strict)"("Blinking"=w1864) -> ()  [unwired: 2 in, 2 out]
                    n1099 = property on="Horizontal Binning 4" class="DigNum (strict)"("Blinking"=w1866) -> ()  [unwired: 2 in, 2 out]
                    n1100 = property on="CCD EM Gain 4" class="DigNum (strict)"("Blinking"=w1861) -> ()  [unwired: 2 in, 2 out]
                    n1101 = property on="Shutter Mode 4" class="Ring (strict)"("Blinking"=w1862) -> ()  [unwired: 2 in, 2 out]
                    n1102 = property on="Shutter TTL 4" class="Ring (strict)"("Blinking"=w1860) -> ()  [unwired: 2 in, 2 out]
                    n1103 = Not(x=w1839) -> (.not. x?=w1854:bool)
                    n1104 = Not(x=w1834) -> (.not. x?=w1857:bool)
                    n1105 = Not(x=w1833) -> (.not. x?=w1855:bool)
                    n1106 = Not(x=w1832) -> (.not. x?=w1856:bool)
                    n1107 = Not(x=w1838) -> (.not. x?=w1858:bool)
                    n1108 = Not(x=w1837) -> (.not. x?=w1836:bool)
                    n1109 = Not(x=w1835) -> (.not. x?=w1859:bool)
                    n1110 = property on="Acquisition Mode 4" class="Ring (strict)"("Blinking"=w1854) -> ()  [unwired: 2 in, 2 out]
                    n1111 = property on="Readout Rate 4" class="Ring (strict)"("Blinking"=w1857) -> ()  [unwired: 2 in, 2 out]
                    n1112 = property on="Vertical Shift Speed 4" class="Ring (strict)"("Blinking"=w1855) -> ()  [unwired: 2 in, 2 out]
                    n1113 = property on="CCD EM Mode 4" class="Ring (strict)"("Blinking"=w1856) -> ()  [unwired: 2 in, 2 out]
                    n1114 = property on="Trigger Mode 4" class="Ring (strict)"("Blinking"=w1858) -> ()  [unwired: 2 in, 2 out]
                    n1115 = property on="Read Mode 4" class="Ring (strict)"("Blinking"=w1836) -> ()  [unwired: 2 in, 2 out]
                    n1116 = property on="Pre-amplification Gain 4" class="Ring (strict)"("Blinking"=w1859) -> ()  [unwired: 2 in, 2 out]
                  }
                }
                n1117 = local write "SI4"(w1779) -> ()
                n1118 = local write "RO4"(w1774) -> ()
                n1119 = local write "PA4"(w1777) -> ()
                n1120 = local write "EA4"(w1778) -> ()
                n1121 = local write "G4"(w1775) -> ()
                n1122 = local write "B4"(w1776) -> ()
                n1123 = local read "Cameras Cluster"() -> (w1827:T7)
                n1124 = Bundle By Name(cluster=w1827, "Current Configuration.Image Initial Line 4"=w1786, "Current Configuration.Image Initial Column 4"=w1784, "Current Configuration.Image Final Line 4"=w1787, "Current Configuration.Image FInal Column 4"=w1785, "Current Configuration.Vertical Binning 4"=w1790, "Current Configuration.Horizontal Binning 4"=w1825, "Current Configuration.Pre-amplification Gain 4"=w1789, "Current Configuration.CCD EM Gain 4"=w1788, "Current Configuration.Readout Rate 4"=w1783, "Current Configuration.Shutter Openning Time 4"=w1824, "Current Configuration.Shutter Closing Time 4"=w1823, "Current Configuration.Vertical Shift Speed 4"=w1822, "Current Configuration.Read Mode 4"=w1821, "Current Configuration.Vertical Clock Voltage 4"=w1820, "Current Configuration.A/D Channel 4"=w1819, "Current Configuration.Shutter Mode 4"=w1814, "Current Configuration.Shutter TTL 4"=w1815, "Current Configuration.Trigger Mode 4"=w1816, "Current Configuration.Frame Transfer 4"=w1817, "Current Configuration.Acquisition Mode 4"=w1818, "Current Configuration.CCD EM Mode 4"=w1782) -> (w1826:T7)
                n1125 = local write "Cameras Cluster"(w1826) -> ()
                n1126 = Compound Arithmetic op=AND(w1797, w1796, w1795, w1794, w1793, w1792, w1791, w1804, w1803, w1802, w1801, w1800, w1799, w1798, w1811, w1810, w1809, w1808, w1807, w1806, w1805) -> (→"CCD checked 4":bool)
                n1127 = property on="Image FInal Column 4" class="DigNum (strict)"("DisabledEnum"=w1772) -> ()  [unwired: 2 in, 2 out]
                n1128 = property on="Frame Transfer 4" class="Bool (strict)"("DisabledEnum"=w1772) -> ()  [unwired: 2 in, 2 out]
                n1129 = property on="Vertical Clock Voltage 4" class="Ring (strict)"("DisabledEnum"=w1772) -> ()  [unwired: 2 in, 2 out]
                n1130 = property on="A/D Channel 4" class="DigNum (strict)"("DisabledEnum"=w1772) -> ()  [unwired: 2 in, 2 out]
                n1131 = property on="Image Initial Line 4" class="DigNum (strict)"("DisabledEnum"=w1772) -> ()  [unwired: 2 in, 2 out]
                n1132 = property on="Image Initial Column 4" class="DigNum (strict)"("DisabledEnum"=w1772) -> ()  [unwired: 2 in, 2 out]
                n1133 = property on="Image Final Line 4" class="DigNum (strict)"("DisabledEnum"=w1772) -> ()  [unwired: 2 in, 2 out]
                n1134 = property on="Shutter Openning Time 4" class="DigNum (strict)"("DisabledEnum"=w1772) -> ()  [unwired: 2 in, 2 out]
                n1135 = property on="Shutter Closing Time 4" class="DigNum (strict)"("DisabledEnum"=w1772) -> ()  [unwired: 2 in, 2 out]
                n1136 = property on="Vertical Binning 4" class="DigNum (strict)"("DisabledEnum"=w1772) -> ()  [unwired: 2 in, 2 out]
                n1137 = property on="Horizontal Binning 4" class="DigNum (strict)"("DisabledEnum"=w1772) -> ()  [unwired: 2 in, 2 out]
                n1138 = property on="Acquisition Mode 4" class="Ring (strict)"("DisabledEnum"=w1772) -> ()  [unwired: 2 in, 2 out]
                n1139 = property on="CCD EM Gain 4" class="DigNum (strict)"("DisabledEnum"=w1772) -> ()  [unwired: 2 in, 2 out]
                n1140 = property on="Shutter Mode 4" class="Ring (strict)"("DisabledEnum"=w1772) -> ()  [unwired: 2 in, 2 out]
                n1141 = property on="Shutter TTL 4" class="Ring (strict)"("DisabledEnum"=w1772) -> ()  [unwired: 2 in, 2 out]
                n1142 = property on="Readout Rate 4" class="Ring (strict)"("DisabledEnum"=w1772) -> ()  [unwired: 2 in, 2 out]
                n1143 = property on="Vertical Shift Speed 4" class="Ring (strict)"("DisabledEnum"=w1772) -> ()  [unwired: 2 in, 2 out]
                n1144 = property on="CCD EM Mode 4" class="Ring (strict)"("DisabledEnum"=w1772) -> ()  [unwired: 2 in, 2 out]
                n1145 = property on="Trigger Mode 4" class="Ring (strict)"("DisabledEnum"=w1772) -> ()  [unwired: 2 in, 2 out]
                n1146 = property on="Read Mode 4" class="Ring (strict)"("DisabledEnum"=w1772) -> ()  [unwired: 2 in, 2 out]
                n1147 = property on="Pre-amplification Gain 4" class="Ring (strict)"("DisabledEnum"=w1772) -> ()  [unwired: 2 in, 2 out]
              }
              frame #19 {
                n1148 = Unbundle By Name(w1938) -> ("object_suffix"=w1937:string, "dflat_suffix"=w1936:string, "sflat_suffix"=w1935:string, "dark_suffix"=w1934:string, "zero_suffix"=w1933:string, "focus_suffix"=w1932:string, "suffixAlertVisible"=w1931:bool)
                n1149 = local write "object suffix"(w1937) -> ()
                n1150 = local write "dflat suffix"(w1936) -> ()
                n1151 = local write "sflat suffix"(w1935) -> ()
                n1152 = local write "dark suffix"(w1934) -> ()
                n1153 = local write "zero suffix"(w1933) -> ()
                n1154 = local write "focus suffix"(w1932) -> ()
                n1155 = property on="suffix alert" class="Str"("Visible"=w1931) -> ()  [unwired: 2 in, 2 out]
                n1156 = case shown="True" w1941 {
                  tunnel: [w1942 w1978] -> w1939
                  tunnel: [w1942 w1962] -> w1940
                  tunnel: w1938 -> [_ w1968]
                  frame False {
                    w1942 = FALSE
                  }
                  frame True {
                    w1948 = TRUE
                    # "Pelo menos 1 canal deve \nestar habilitado"
                    n1157 = local read "Preview Temp."() -> (w1967:dbl)
                    n1158 = Unbundle By Name(w1968) -> ("ChannelA_Status.target  temp"=w1964:i16, "ChannelB_Status.target  temp"=w1966:i16, "ChannelC_Status.target  temp"=w1965:i16, "ChannelD_Status.target  temp"=w1963:i16)
                    n1159 = property on="CCD checked 3" class="Bool (strict)"() -> ("Value"=w1974:bool)  [unwired: 2 in, 2 out]
                    n1160 = local read "CH3 on"() -> (w1958:bool)
                    n1161 = local read "CH1on"() -> (w1960:bool)
                    n1162 = property on="CCD checked 2" class="Bool (strict)"() -> ("Value"=w1977:bool)  [unwired: 2 in, 2 out]
                    n1163 = local read "CH2on"() -> (w1959:bool)
                    n1164 = property on="CCD checked 1" class="Bool (strict)"() -> ("Value"=w1981:bool)  [unwired: 2 in, 2 out]
                    n1165 = property on="CCD checked 4" class="Bool (strict)"() -> ("Value"=w1971:bool)  [unwired: 2 in, 2 out]
                    n1166 = local read "CH4 on"() -> (w1957:bool)
                    n1167 = To Word Integer(number=w1967) -> (16bit integer=w1961:i16)
                    n1168 = Select(t=w1981, s=w1960, f=TRUE) -> (s? t:f=w1979:bool)
                    n1169 = local read "CH3 on"() -> (w1950:bool)
                    n1170 = local read "CH4 on"() -> (w1949:bool)
                    n1171 = Compound Arithmetic op=OR(w1960, w1959, w1958, w1957) -> (w1947:bool)
                    n1172 = local read "CH2on"() -> (w1951:bool)
                    n1173 = Select(t=w1974, s=w1958, f=TRUE) -> (s? t:f=w1972:bool)
                    n1174 = Select(t=w1977, s=w1959, f=TRUE) -> (s? t:f=w1975:bool)
                    n1175 = Select(t=w1971, s=w1957, f=TRUE) -> (s? t:f=w1969:bool)
                    n1176 = Equal?(x=w1961, y=w1966) -> (x = y?=w1955:bool)
                    n1177 = Equal?(x=w1961, y=w1965) -> (x = y?=w1954:bool)
                    n1178 = Equal?(x=w1961, y=w1963) -> (x = y?=w1953:bool)
                    n1179 = Equal?(x=w1961, y=w1964) -> (x = y?=w1956:bool)
                    n1180 = local read "CH1on"() -> (w1952:bool)
                    n1181 = Select(t=w1956, s=w1952, f=w1948) -> (s? t:f=w1946:bool)
                    n1182 = Select(t=w1954, s=w1950, f=w1948) -> (s? t:f=w1944:bool)
                    n1183 = Select(t=w1953, s=w1949, f=w1948) -> (s? t:f=w1943:bool)
                    n1184 = Select(t=w1955, s=w1951, f=w1948) -> (s? t:f=w1945:bool)
                    n1185 = Compound Arithmetic op=AND(w1979, w1975, w1972, w1969, w1947) -> (w1978:bool)
                    n1186 = Compound Arithmetic op=AND(w1947, w1946, w1945, w1944, w1943) -> (w1962:bool)
                  }
                }
                "SET Temp status" <- w1940
                "SET CCD status" <- w1939
              }
            }
            n1187 = call-dynamic "Read Obs_state.vi"("error in (no error)"=w325, "S4ACS_GUI in"=w326) -> ("error out"=w302:errorcluster, "Obs_state"=w322:u32, "S4ACS_GUI out"=w303:refnum<class "S4GUI.lvclass">)  [unwired: 7 in]
            n1188 = In Range and Coerce(upper limit=u32 226, x=w322, lower limit=u32 220 ("upper limit")) -> (In Range?=w320:bool)  [unwired: 1 out]
